vi "Get Message Parameters.vi"(8 "error in (no error)":errorcluster, 11 "Message ref in":u64) -> (0 "error out":errorcluster, 2 "Message Metadata":T1, 3 "Message ref out":u64)   [LabVIEW 2019, in "gRPC Template Creation Utility.lvlib"]
uses:
  gRPC Template Creation Utility.lvlib
  TypeDefs/Message Metadata (Scripting).ctl
  TypeDefs/Message Element Metadata (Scripting).ctl
  TypeDefs/Message Element Type.ctl
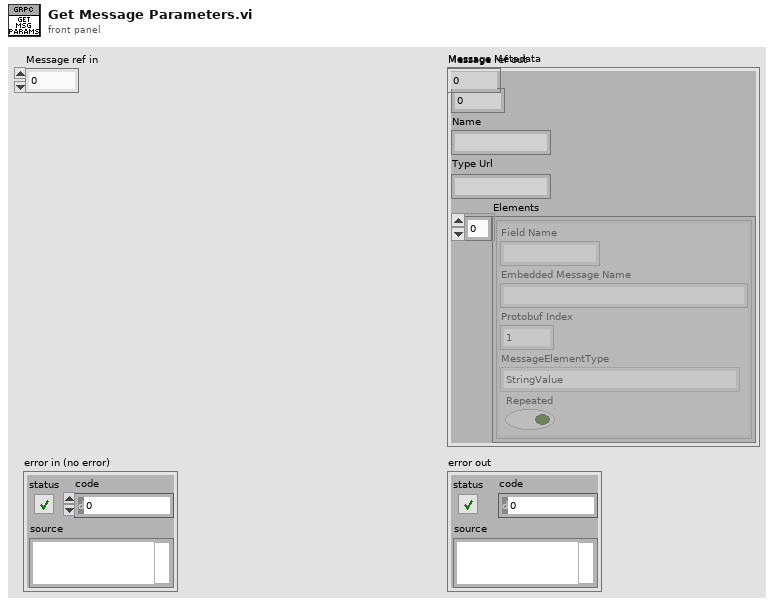
[diagram p1: front panel]
types:
  T1 = typedef "gRPC Template Creation Utility.lvlib/Message Metadata (Scripting).ctl" = cluster{"Version":i32, "Name":string, "Type Url":string, "Elements":T2[]}
  T2 = typedef "gRPC Template Creation Utility.lvlib/Message Element Metadata (Scripting).ctl" = cluster{"Field Name":string, "Embedded Message Name":string, "Protobuf Index":i32, "MessageElementType":T3, "Repeated":bool}
  T3 = typedef "gRPC Template Creation Utility.lvlib/Message Element Type.ctl" = enum32{"Int32Value", "FloatValue", "DoubleValue", "BoolValue", "StringValue", "MessageValue", "Int64Value", "UInt32Value", "UInt64Value", "EnumValue", "Bytes", "Fixed64", "Fixed32", "SFixed64", "SFixed32", "SInt64", "SInt32"}
  T4 = typedef "gRPC Scripting Tools.lvlib/Message Element Metadata (Scripting).ctl" = cluster{"Field Name":string, "Embedded Message Name":string, "Protobuf Index":i32, "MessageElementType":T5, "Repeated":bool}
  T5 = typedef "gRPC Scripting Tools.lvlib/Message Element Type.ctl" = enum32{"Int32Value", "FloatValue", "DoubleValue", "BoolValue", "StringValue", "MessageValue", "Int64Value", "UInt32Value", "UInt64Value", "EnumValue", "Bytes", "Fixed64", "Fixed32", "SFixed64", "SFixed32", "SInt64", "SInt32"}
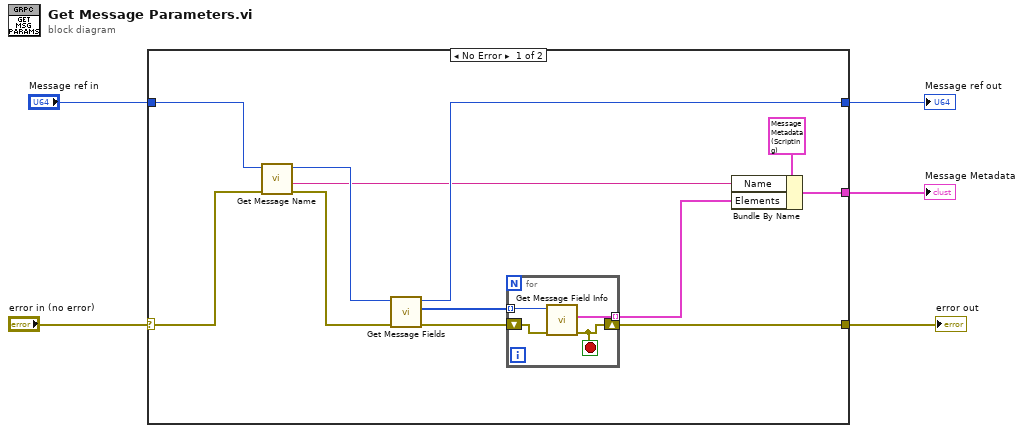
[diagram p0: block diagram]
diagram:
  n1 = case shown="No Error" "error in (no error)" {
    selector: "error in (no error)" -> [w9 w23]
    tunnel: "Message ref in" -> [w12 w22]
    tunnel: [w11 _] -> w4
    tunnel: [w10 w22] -> w3
    tunnel: [w7 w23] -> w1
    frame No Error {
      n2 = call "Get Message Name.vi"("error in (no error)"=w9, "Message ref in"=w12) -> ("error out"=w17:errorcluster, "Message Name"=w6:string, "Message ref out"=w16:u64)  [unwired: 7 in]
      n3 = call "Get Message Fields.vi"("error in (no error)"=w17, "Message ref in"=w16) -> ("error out"=w8:errorcluster, "Field refs"=w13:u64[], "Message ref out"=w10:u64)  [unwired: 7 in]
      n4 = for {
        tunnel: w13 -> [w21] mode=indexing
        tunnel: [w20] -> w14 mode=indexing
        shift-right: [w18] -> w7
        shift-left: w8 -> [w19]
        stop <- w18 stop-if-true
        n5 = call "Get Message Field Info.vi"("error in (no error)"=w19, "Message Field ref in"=w21) -> ("error out"=w18:errorcluster, "Field Info"=w20:T4)  [unwired: 7 in, 1 out]
      }
      n6 = Bundle By Name(cluster=T1 {"Version"=0, "Name"="InvokeRequest", "Type Url"="", "Elements"=[{"Field Name"="command", "Embedded Message Name"="", "Protobuf Index"=1, "MessageElementType"=enum."StringValue", "Repeated"=FALSE}, {"Field Name"="parameter", "Embedded Message Name"="", "Protobuf Index"=2, "MessageElementType"=enum."StringValue", "Repeated"=FALSE}]} ("Message Metadata"), "Name"=w6, "Elements"=w14) -> (w11:T1)
    }
    frame Error {
    }
  }
  "Message Metadata" <- w4
  "Message ref out" <- w3
  "error out" <- w1
